vi "Unique_Selector_Values.vi"(3 "Precision":string, 4 "Bin Centres":dbl[](array[numeric]) format="%.4f") -> (1 "Bin Strings":string[](array[string]))   [LabVIEW 2021]
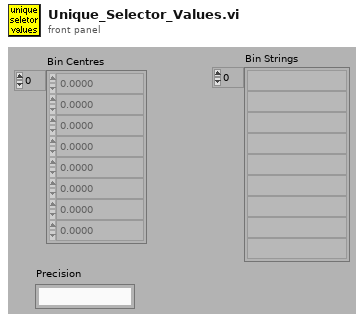
[diagram p1: front panel]
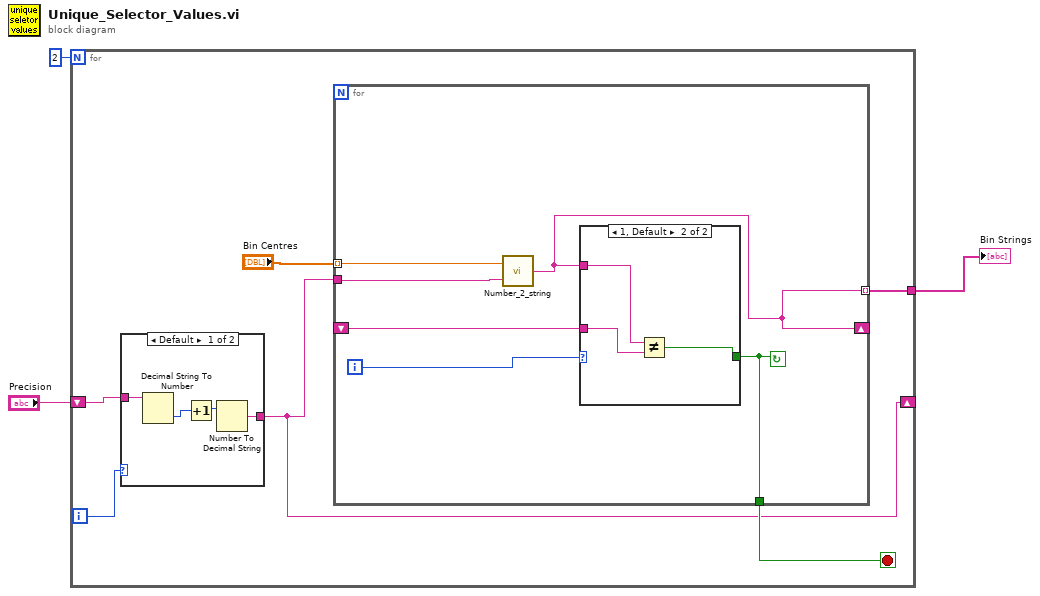
[diagram p0: block diagram]
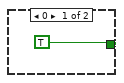
[diagram p3: hidden frame]
diagram:
  n1 = for {
    N: 2 -> [_]
    tunnel: [w8] -> w3
    shift-right: [w4] -> _
    shift-left: "Precision" -> [w7]
    i -> [w6]
    stop <- w5 stop-if-true
    n2 = case shown="Default" w6 {
      tunnel: w7 -> [w13 w14]
      tunnel: [w10 w14] -> w4
      frame Default {
        n3 = Decimal String To Number(string=w13) -> (number=w12:i32)  [unwired: 3 out]
        n4 = Increment(x=w12) -> (x+1=w11:i32)
        n5 = Number To Decimal String(number=w11) -> (decimal integer string=w10:string)  [unwired: 1 out]
      }
      frame 0 {
      }
    }
    n6 = for {
      tunnel: "Bin Centres" -> [w16] mode=indexing
      tunnel: w4 -> [w18]
      shift-right: [w17] -> _
      shift-left: _ -> [w19]
      tunnel: [w17] -> w8 mode=indexing
      tunnel: [w15] -> w5
      i -> [w20]
      stop <- w15 continue-if-true
      n7 = call "Number_2_string.vi"("precision"=w18, "number"=w16) -> ("String"=w17:string)
      n8 = case shown="1, Default" w20 {
        tunnel: w17 -> [_ w24]
        tunnel: w19 -> [_ w23]
        tunnel: [TRUE w22] -> w15
        frame 0 {
        }
        frame 1, Default {
          n9 = Not Equal?(x=w24, y=w23) -> (x != y?=w22:bool)
        }
      }
    }
  }
  "Bin Strings" <- w3
